vi "Flatten.vi"(8 "error in (no error)":errorcluster, 9 "Attributes":string[](array[string]), 10 "Pretty Print?":bool, 11 "JSON Value in":refnum<class "JSON Value.lvclass">) -> (0 "error out":errorcluster, 2 "String":string)   [LabVIEW 2011, in "JSON Value.lvclass"]
uses:
  JSON Value.lvclass
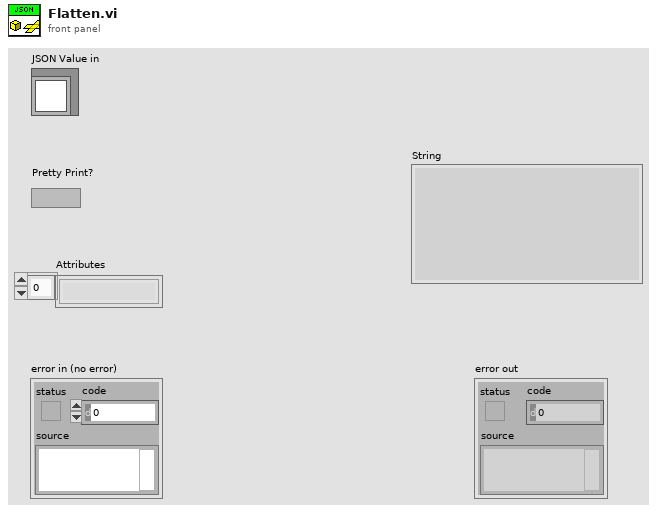
[diagram p1: front panel]
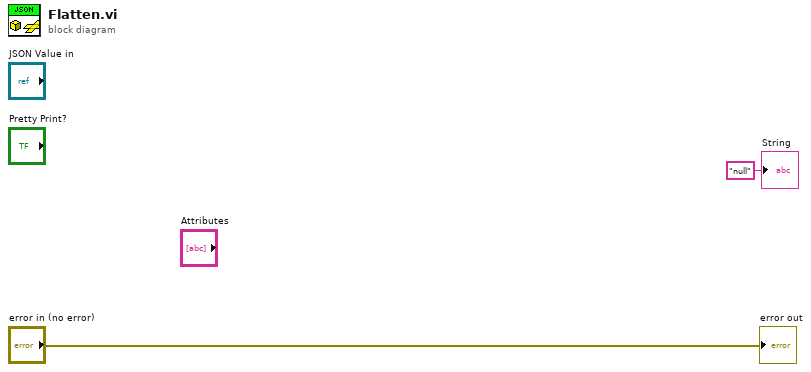
[diagram p0: block diagram]
diagram:
  "error out" <- "error in (no error)"
  "String" <- "null" ("String")
